vi "Current Time.vi"(8 "error in (no error)":errorcluster, 11 "Model in":refnum<class "Model.lvclass">) -> (0 "error out":errorcluster, 2 "Time":dbl, 3 "Model out":refnum<class "Model.lvclass">)   [LabVIEW 2016, in "Model.lvclass"]
uses:
  Model.lvclass
  Model.lvclass/Model.ctl
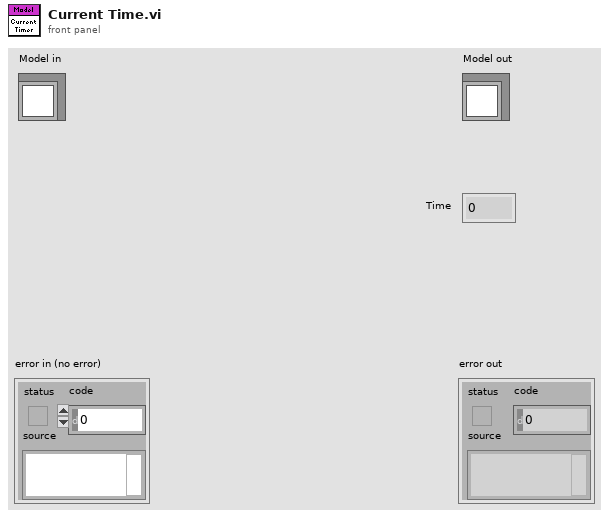
[diagram p1: front panel]
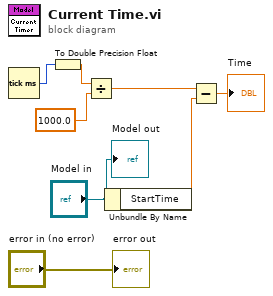
[diagram p0: block diagram]
diagram:
  n1 = Tick Count (ms)() -> (millisecond timer value=w2:u32)
  n2 = To Double Precision Float(number=w2) -> (double precision float=w1:dbl)
  n3 = Divide(x=w1, y=1000.0) -> (x/y=w3:dbl)
  n4 = Unbundle By Name("Model in") -> ("StartTime"=w8:dbl)
  n5 = Subtract(x=w3, y=w8) -> (x-y=→"Time":dbl)
  "error out" <- "error in (no error)"
  "Model out" <- "Model in"
